vi "CRIS Value Relay.vi"() -> ()   [LabVIEW 2013]
panel:
  in  "Update Rate (milliseconds)":u32=10
  out "Loop Counter":i32
  in  "Stop Button":bool
  out "isNew":bool
  in  "isOK":bool
  out "waveSet":dbl
  in  "waveReadback":dbl
  # "CRIS writes through Python"
  # "CRIS reads through Python"
  # "These controls are configured as indicators with data binding enabled. They link to the RILIS VM shared variables, relaying values written by python to the local project shared variables to the remote RILIS shared variables."
  # "These indicators are configured as controls with data binding enabled. They link to the RILIS VM shared variables, relaying values written remotely by RILIS to the local project shared variables read by python."
  # "These controls and indicators are set to 'disabled' to prevent accidently changing a value here. This VI just acts as a relay."
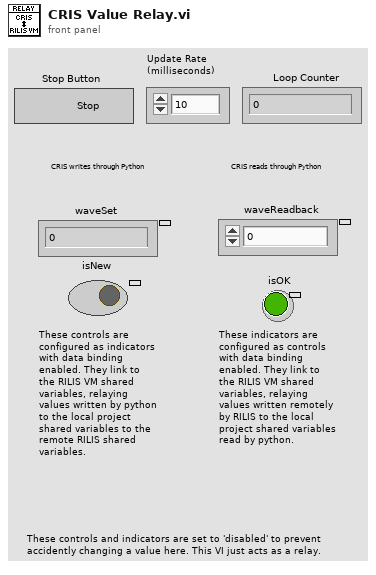
[diagram p1: front panel]
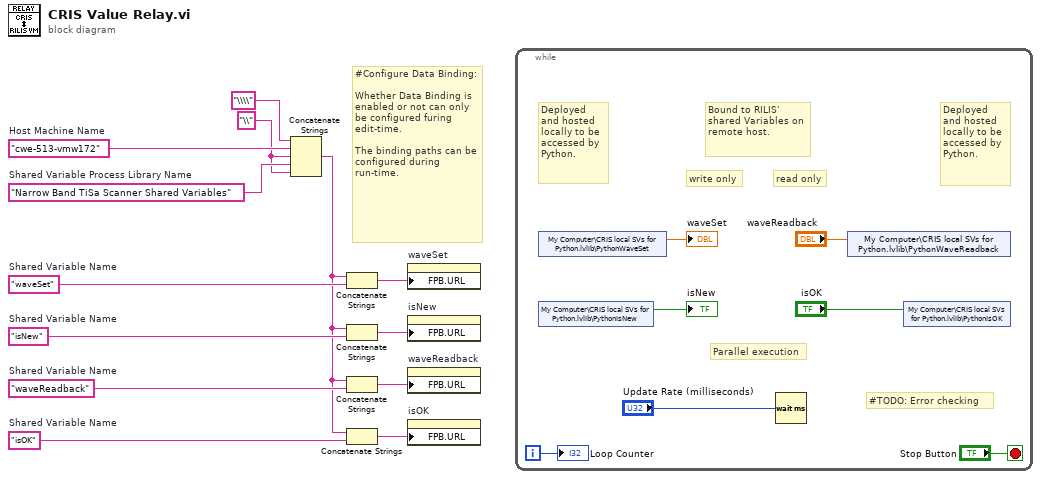
[diagram p0: block diagram]
diagram:
  w10 = "\\"
  w9 = "waveSet"  # Shared Variable Name
  w3 = "waveReadback"  # Shared Variable Name
  w2 = "isOK"  # Shared Variable Name
  w11 = "Narrow Band TiSa Scanner Shared Variables"  # Shared Variable Process Library Name
  w4 = "isNew"  # Shared Variable Name
  w12 = "cwe-513-vmw172"  # Host Machine Name
  # "#Configure Data Binding:\n\nWhether Data Binding is enabled or not can only be configured furing edit-time.\n\nThe binding paths can be configured during run-time."
  n1 = Concatenate Strings("\\\\", w12, w10, w11, w10) -> (w1:string)
  n2 = Concatenate Strings(w1, w9) -> (w8:string)
  n3 = Concatenate Strings(w1, w4) -> (w7:string)
  n4 = Concatenate Strings(w1, w3) -> (w6:string)
  n5 = Concatenate Strings(w1, w2) -> (w5:string)
  n6 = property on="waveSet" class="DigNum (strict)"("FPB.URL"=w8) -> ()  [unwired: 2 in, 2 out]
  n7 = property on="isNew" class="Bool (strict)"("FPB.URL"=w7) -> ()  [unwired: 2 in, 2 out]
  n8 = property on="waveReadback" class="DigNum (strict)"("FPB.URL"=w6) -> ()  [unwired: 2 in, 2 out]
  n9 = property on="isOK" class="Bool (strict)"("FPB.URL"=w5) -> ()  [unwired: 2 in, 2 out]
  n10 = while {
    i -> [w19]
    stop <- "Stop Button" stop-if-true
    # "Parallel execution"
    # "#TODO: Error checking"
    # "Deployed and hosted locally to be accessed by Python."
    # "Deployed and hosted locally to be accessed by Python."
    # "read only"
    # "write only"
    # "Bound to RILIS' shared Variables on remote host."
    n11 = shared-variable "My Computer\\CRIS local SVs for Python.lvlib\\PythonWaveSet"() -> (→"waveSet":dbl)  [unwired: 1 in, 1 out]
    n12 = shared-variable "My Computer\\CRIS local SVs for Python.lvlib\\PythonIsNew"() -> (→"isNew":bool)  [unwired: 1 in, 1 out]
    n13 = Wait (ms)(milliseconds to wait="Update Rate (milliseconds)") -> ()  [unwired: 1 out]
    n14 = shared-variable "My Computer\\CRIS local SVs for Python.lvlib\\PythonWaveReadback"("waveReadback") -> ()  [unwired: 1 in, 1 out]
    n15 = shared-variable "My Computer\\CRIS local SVs for Python.lvlib\\PythonIsOK"("isOK") -> ()  [unwired: 1 in, 1 out]
    "Loop Counter" <- w19
  }
